vi "Autonomous Independent.vi"   [LabVIEW 2017]
doc: "This VI is called when autonomous begins, and will automatically be terminated when autonomous ends. You can carry out timed or sensor driven robot movement independently without needing to return to the caller."
uses:
  Public/Documents/Cross The Road Electronics/Phoenix-LabVIEW/Motor Controller/Controls/CTRE_Phoenix_MotorControl_ControlMode.ctl
  <vilib>/Rock Robotics/WPI/Utilities/WPI_GetSetVariantRefNum.vi
  <vilib>/Rock Robotics/Network Tables/NT Read String.vi
  <vilib>/Rock Robotics/Network Tables/NT Write Numeric Array.vi
panel:
  # "Be sure to right-click and choose Data Operations>>Make Current Value default if you want to save the array values with the VI"
types:
  T1 = typedef "WPI_RobotDriveDevRef.ctl" = cluster{"DevStatus":errorcluster, "Motors[]":T2[], "Square Inputs":bool, "Max Output":dbl}
  T2 = typedef "WPI_MotorControlDeviceRef.ctl" = cluster{"DeviceStatus":errorcluster, "Type":T3, "PWM":cluster{"PWM Channel":T4, "DeadBand":T5}, "CAN":cluster{"Device Number":u8, "SetOutput VI Ref":variant, "GetOutput VI Ref":variant, "Enable VI Ref":variant, "Disable VI Ref":variant, "Data":variant}, "Invert":bool, "DIO PWM":cluster{"PWM \"Enable\" Channel":T4, "DIOChannel":T6, "PWM Rate":dbl}}
  T3 = typedef "WPI_MotorControlType.ctl" = enum16{"PWM", "CAN", "DIO PWM"}
  T4 = typedef "FPGA_DIOPWMChannel.ctl" = enum8{"PWM 0", "PWM 1", "PWM 2", "PWM 3", "PWM 4", "PWM 5", "PWM 6", "PWM 7", "PWM 8", "PWM 9", "PWM MXP 0", "PWM MXP 1", "PWM MXP 2", "PWM MXP 3", "PWM MXP 4", "PWM MXP 5", "PWM MXP 6", "PWM MXP 7", "PWM MXP 8", "PWM MXP 9", "Invalid"}
  T5 = typedef "WPI_PWMDeadband.ctl" = cluster{"Name":string, "maxPositivePwm":i32, "minPositivePwm":i32, "centerPwm":i32, "maxNegativePwm":i32, "minNegativePwm":i32, "angularRange":u16}
  T6 = typedef "FPGA_DIOChannel.ctl" = enum8{"DIO 0", "DIO 1", "DIO 2", "DIO 3", "DIO 4", "DIO 5", "DIO 6", "DIO 7", "DIO 8", "DIO 9", "DIO MXP 0", "DIO MXP 1", "DIO MXP 2", "DIO MXP 3", "DIO MXP 4", "DIO MXP 5", "DIO MXP 6", "DIO MXP 7", "DIO MXP 8", "DIO MXP 9", "DIO MXP 10", "DIO MXP 11", "DIO MXP 12", "DIO MXP 13", "DIO MXP 14", "DIO MXP 15", "SPI Port CS1", "SPI Port CS2", "SPI Port CS3", "SPI Port MISO", "SPI Port MOSI", "Invalid"}
  T7 = typedef "WPI_JoystickDevRef.ctl" = cluster{"Device":T8}
  T8 = typedef "WPI_JoystickDeviceEnum.ctl" = enum16{"USB 0", "USB 1", "USB 2", "USB 3", "USB 4", "USB 5"}
  T9 = typedef "CTRE_Phoenix_MotorControl_ControlMode.ctl" = u16
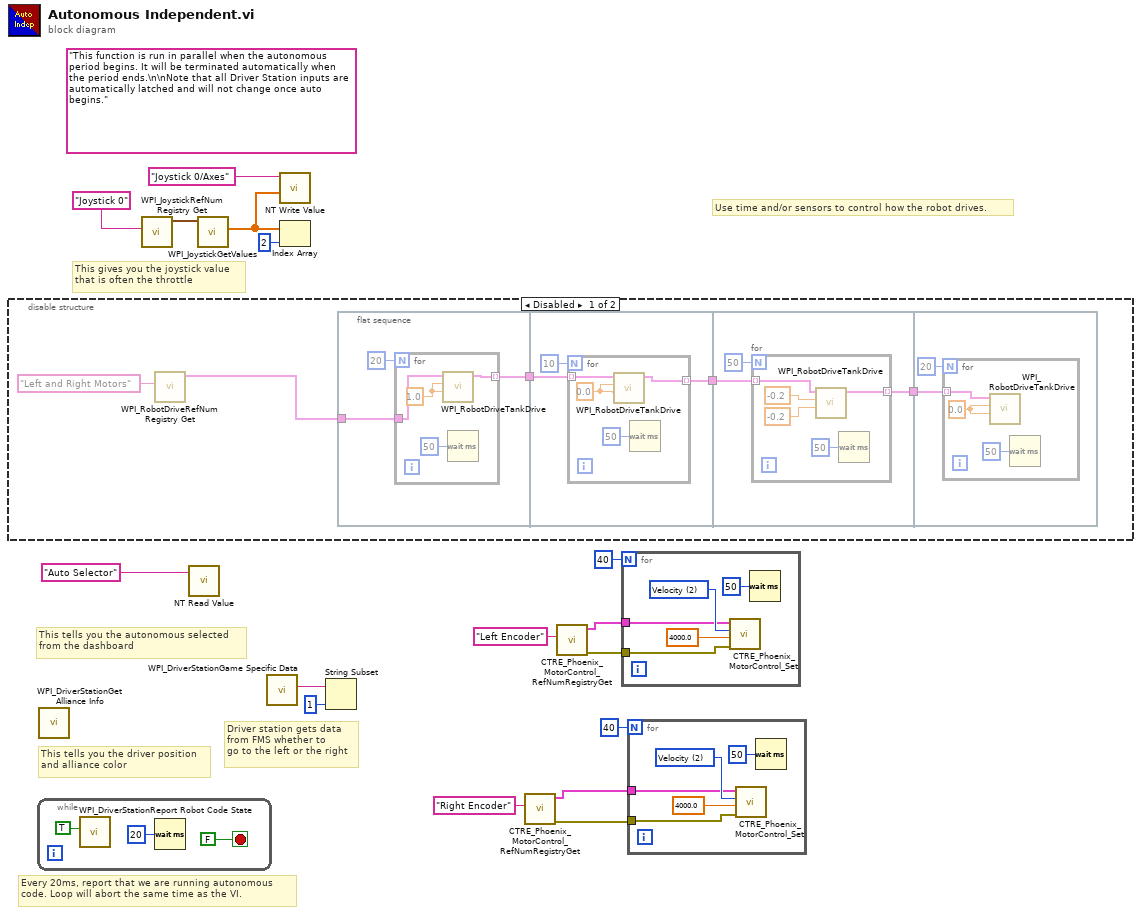
[diagram p0: block diagram]
diagram:
  (unwired) "This function is run in parallel when the autonomous period begins. It will be terminated automatically when the period ends.\n\nNote that all Driver Station inputs are automatically latched and will not change once auto begins."
  # "Driver station gets data \nfrom FMS whether to\ngo to the left or the right"
  # "This tells you the autonomous selected\nfrom the dashboard"
  # "Every 20ms, report that we are running autonomous\ncode. Loop will abort the same time as the VI."
  # "This gives you the joystick value\nthat is often the throttle"
  # "Use time and/or sensors to control how the robot drives."
  # "This tells you the driver position\nand alliance color"
  n1 = disable-structure shown="Disabled" {
    frame Disabled {
      n2 = call <vilib>:"WPI_RobotDriveRefNum Registry Get.vi"("refnum name"="Left and Right Motors") -> ("RobotDriveDevRef"=w17:T1)  [unwired: 9 in, 1 out]
      n3 = flat-sequence {
        tunnel: w17 -> [w24]
        tunnel: [w22] -> w21
        tunnel: w21 -> [w31]
        tunnel: [w29] -> w20
        tunnel: w20 -> [w37]
        tunnel: [w36] -> w19
        tunnel: w19 -> [w45]
        frame #0 {
          n4 = for {
            N: 20 -> [_]
            tunnel: w24 -> [w27]
            tunnel: [w25] -> w22 mode=indexing
            w28 = 1.0 ("Right axis value")
            n5 = call <vilib>:"WPI_RobotDriveTankDrive.vi"("Right axis value"=w28, "Left axis value"=w28, "RobotDriveDevRef"=w27) -> ("RobotDriveDevRef"=w25:T1)  [unwired: 6 in, 2 out]
            n6 = Wait (ms)(milliseconds to wait=u32 50) -> ()  [unwired: 1 out]
          }
        }
        frame #1 {
          n7 = for {
            N: 10 -> [_]
            tunnel: w31 -> [w35] mode=indexing
            tunnel: [w32] -> w29 mode=indexing
            w34 = 0.0 ("Left axis value")
            n8 = call <vilib>:"WPI_RobotDriveTankDrive.vi"("Right axis value"=w34, "Left axis value"=w34, "RobotDriveDevRef"=w35) -> ("RobotDriveDevRef"=w32:T1)  [unwired: 6 in, 2 out]
            n9 = Wait (ms)(milliseconds to wait=u32 50) -> ()  [unwired: 1 out]
          }
        }
        frame #2 {
          n10 = for {
            N: 50 -> [_]
            tunnel: w37 -> [w40] mode=indexing
            tunnel: [w39] -> w36 mode=indexing
            n11 = call <vilib>:"WPI_RobotDriveTankDrive.vi"("Right axis value"=-0.2, "Left axis value"=-0.2, "RobotDriveDevRef"=w40) -> ("RobotDriveDevRef"=w39:T1)  [unwired: 6 in, 2 out]
            n12 = Wait (ms)(milliseconds to wait=u32 50) -> ()  [unwired: 1 out]
          }
        }
        frame #3 {
          n13 = for {
            N: 20 -> [_]
            tunnel: w45 -> [w47] mode=indexing
            w48 = 0.0 ("Left axis value")
            n14 = call <vilib>:"WPI_RobotDriveTankDrive.vi"("Right axis value"=w48, "Left axis value"=w48, "RobotDriveDevRef"=w47) -> ()  [unwired: 6 in, 3 out]
            n15 = Wait (ms)(milliseconds to wait=u32 50) -> ()  [unwired: 1 out]
          }
        }
      }
    }
    frame Enabled {
    }
  }
  n16 = while {
    stop <- FALSE stop-if-true
    n17 = call <vilib>:"WPI_DriverStationReport Robot Code State.vi"("Autonomous"=TRUE) -> ()  [unwired: 10 in, 1 out]
    n18 = Wait (ms)(milliseconds to wait=u32 20) -> ()  [unwired: 1 out]
  }
  n19 = call <vilib>:"WPI_DriverStationGet Alliance Info.vi"() -> ()  [unwired: 12 out]
  n20 = call <vilib>:"WPI_JoystickRefNum Registry Get.vi"("refnum name"="Joystick 0") -> ("JoystickDevRef"=w15:T7)  [unwired: 1 in, 9 out]
  n21 = call-poly <vilib>:"NT Read Value.vi"("Name"="Auto Selector") -> ()  [unwired: 9 in, 2 out]
  n22 = call <vilib>:"WPI_JoystickGetValues.vi"("JoystickDevRef"=w15) -> ("Axes"=w12:dbl[])  [unwired: 6 in, 4 out]
  n23 = call <vilib>:"WPI_DriverStationGame Specific Data.vi"() -> ("Game Specific Data"=w8:string)  [unwired: 11 in]
  n24 = call-poly <vilib>:"NT Write Value.vi"("Numeric Array"=w12, "Name"="Joystick 0/Axes") -> ()  [unwired: 9 in, 1 out]
  n25 = Index Array(array=w12, index=2) -> ()  [unwired: 1 out]
  n26 = String Subset(string=w8, length (rest)=1 ("length (rest)")) -> ()  [unwired: 1 in, 1 out]
  n27 = call <vilib>:"CTRE_Phoenix_MotorControl_RefNumRegistryGet.vi"("refnum name"="Right Encoder") -> ("error out"=w2:errorcluster, "PhoenixMotorControlDevRef"=w3:T2)  [unwired: 9 in]
  n28 = call <vilib>:"CTRE_Phoenix_MotorControl_RefNumRegistryGet.vi"("refnum name"="Left Encoder") -> ("error out"=w5:errorcluster, "PhoenixMotorControlDevRef"=w6:T2)  [unwired: 9 in]
  n29 = for {
    N: 40 -> [_]
    tunnel: w6 -> [w54]
    tunnel: w5 -> [w53]
    w56 = T9 2 items=["PercentOutput"=0, "Position"=1, "Velocity"=2, "Current"=3, "Follower"=5, "MotionProfile"=6, "MotionMagic"=7, "MotionMagicArc"=8, "MotionProfileArc"=10, "Disabled"=15] ("Control Mode")
    n30 = call <vilib>:"CTRE_Phoenix_MotorControl_Set.vi"("error in (no error)"=w53, "Output"=4000.0, "Control Mode"=w56, "PhoenixMotorControlDevRef"=w54) -> ()  [unwired: 6 in, 2 out]
    n31 = Wait (ms)(milliseconds to wait=u32 50) -> ()  [unwired: 1 out]
  }
  n32 = for {
    N: 40 -> [_]
    tunnel: w3 -> [w59]
    tunnel: w2 -> [w58]
    w61 = T9 2 items=["PercentOutput"=0, "Position"=1, "Velocity"=2, "Current"=3, "Follower"=5, "MotionProfile"=6, "MotionMagic"=7, "MotionMagicArc"=8, "MotionProfileArc"=10, "Disabled"=15] ("Control Mode")
    n33 = call <vilib>:"CTRE_Phoenix_MotorControl_Set.vi"("error in (no error)"=w58, "Output"=4000.0, "Control Mode"=w61, "PhoenixMotorControlDevRef"=w59) -> ()  [unwired: 6 in, 2 out]
    n34 = Wait (ms)(milliseconds to wait=u32 50) -> ()  [unwired: 1 out]
  }
